vi "Area_Of_A_Trapezium.vi"() -> ()   [LabVIEW 2014]
panel:
  in  "Height":dbl
  in  "Length B":dbl
  in  "Length A":dbl
  in  "Calculate":bool
  out "Result":dbl
  # "A calculator for working out the area of a trapezium"
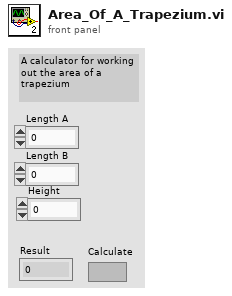
[diagram p1: front panel]
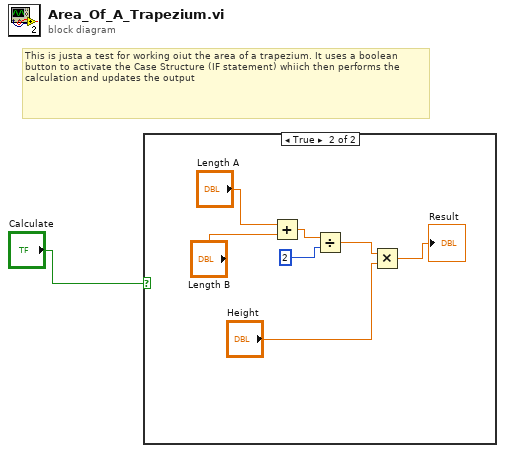
[diagram p0: block diagram]
diagram:
  # "This is justa a test for working oiut the area of a trapezium. It uses a boolean button to activate the Case Structure (IF statement) whiich then performs the calculation and updates the output"
  n1 = case shown="True" "Calculate" {
    frame False {
    }
    frame True {
      n2 = Add(x="Length A", y="Length B") -> (x+y=w8:dbl)
      n3 = Divide(x=w8, y=2) -> (x/y=w2:dbl)
      n4 = Multiply(x=w2, y="Height") -> (x*y=→"Result":dbl)
    }
  }
